vi "motor_choose_step.vi"(8 "error In":errorcluster, 9 "JSON string":string, 10 "Step order":string, 11 "process_ID":string) -> (0 "error IO":errorcluster)   [LabVIEW 2020]
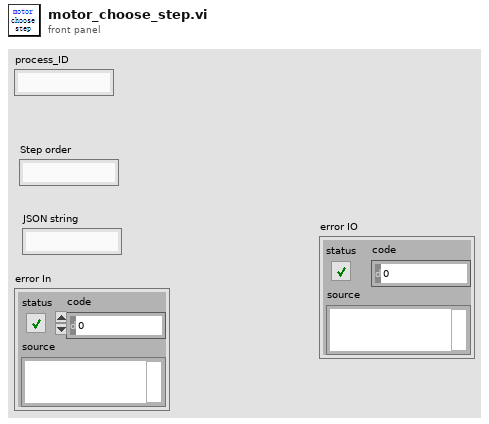
[diagram p1: front panel]
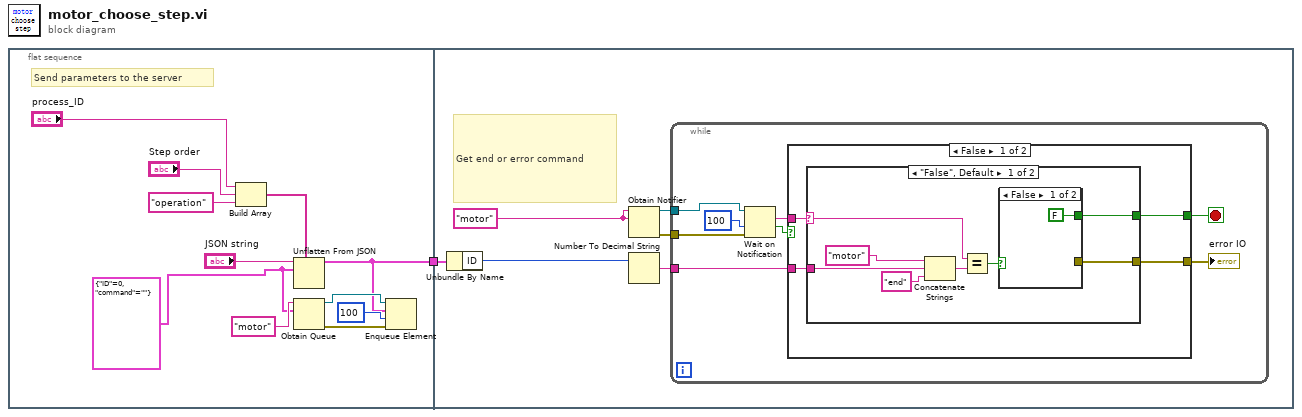
[diagram p0: block diagram]
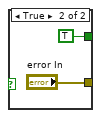
[diagram p2: hidden frame]
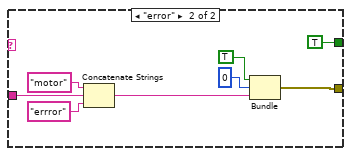
[diagram p3: hidden frame]
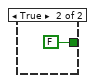
[diagram p4: hidden frame]
diagram:
  n1 = flat-sequence {
    tunnel: [w4] -> w1
    tunnel: w1 -> [w15]
    frame #0 {
      w2 = cluster{"ID":i32, "command":string} {"ID"=0, "command"=""} ("参数")
      # "Send parameters to the server"
      n2 = Build Array("process_ID", "Step order", "operation" ("string")) -> (w10:string[])
      n3 = Unflatten From JSON(path=w10, JSON string="JSON string", type and defaults=w2) -> (value=w4:cluster{"ID":i32, "command":string})  [unwired: 4 in, 1 out]
      n4 = Obtain Queue(name (unnamed)="motor", element data type=w2) -> (queue out=w11:refnum<queue>, error out=w12:errorcluster)  [unwired: 3 in, 1 out]
      n5 = Enqueue Element(queue=w11, element=w4, timeout in ms (-1)=100, error in (no error)=w12) -> ()  [unwired: 3 out]
    }
    frame #1 {
      w16 = "motor" ("name (unnamed)")
      # "Get end or error command"
      n6 = Unbundle By Name(w15) -> ("ID"=w14:i32)
      n7 = Obtain Notifier(name (unnamed)=w16, notification data type=w16) -> (notifier out=w18:refnum<notifier>, error out=w17:errorcluster)  [unwired: 2 in, 1 out]
      n8 = Number To Decimal String(number=w14) -> (decimal integer string=w13:string)  [unwired: 1 in]
      n9 = while {
        tunnel: w18 -> [w26]
        tunnel: w17 -> [w23]
        tunnel: w13 -> [w20]
        stop <- w21 stop-if-true
        n10 = Wait on Notification(notifier=w26, timeout in ms (-1)=100, error in (no error)=w23) -> (notification=w22:string, timed out?=w24:bool)  [unwired: 1 in, 2 out]
        n11 = case shown="False" w24 {
          tunnel: w22 -> [w30 _]
          tunnel: [w29 FALSE] -> w21
          tunnel: w20 -> [w28 _]
          tunnel: [w27 _] -> w19
          frame False {
            n12 = case shown="\"False\", Default" w30 {
              selector: w30 -> [w38 _]
              tunnel: [w36 TRUE] -> w29
              tunnel: [w31 w46] -> w27
              tunnel: w28 -> [w35 w42]
              frame "False", Default {
                n13 = Concatenate Strings("motor" ("string"), w35, "end" ("string")) -> (w33:string)
                n14 = Equal?(x=w38, y=w33) -> (x = y?=w37:bool)
                n15 = case shown="False" w37 {
                  tunnel: [FALSE TRUE] -> w36
                  tunnel: [_ "error In"] -> w31
                  frame False {
                  }
                  frame True {
                  }
                }
              }
              frame "error" {
                n16 = Concatenate Strings("motor" ("string"), w42, "errror" ("string")) -> (w43:string)
                n17 = Bundle("status"=TRUE, "code"=0, w43) -> (w46:cluster{"status":bool, "code":i32, string})  [unwired: 1 in]
              }
            }
          }
          frame True {
          }
        }
        "error IO" <- w19
      }
    }
  }
